vi "Scale.vi"(10 "Params":T1(array[cluster]), 11 "Frequences":dbl[](array[numeric])) -> (3 "ScaleFrequences":dbl[](array[numeric]))   [LabVIEW 2024]
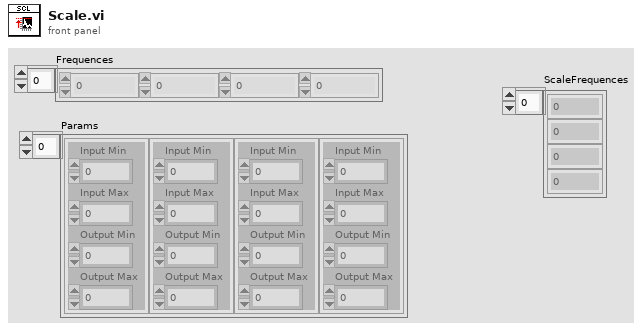
[diagram p1: front panel]
types:
  T1 = cluster{"Input Min":dbl, "Input Max":dbl, "Output Min":dbl, "Output Max":dbl}[]
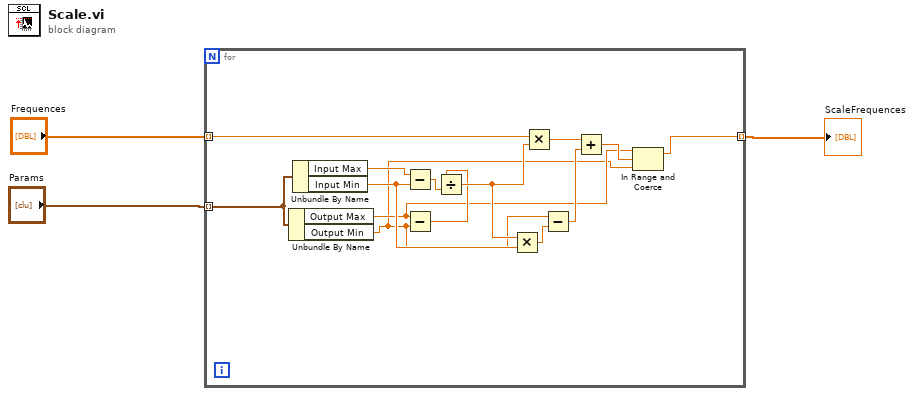
[diagram p0: block diagram]
diagram:
  n1 = for {
    tunnel: "Params" -> [w10] mode=indexing
    tunnel: "Frequences" -> [w11] mode=indexing
    tunnel: [w13] -> w1 mode=indexing
    n2 = Unbundle By Name(w10) -> ("Output Max"=w5:dbl, "Output Min"=w4:dbl)
    n3 = Unbundle By Name(w10) -> ("Input Max"=w12:dbl, "Input Min"=w6:dbl)
    n4 = Subtract(x=w12, y=w6) -> (x-y=w8:dbl)
    n5 = Subtract(x=w5, y=w4) -> (x-y=w7:dbl)
    n6 = Divide(x=w7, y=w8) -> (x/y=w9:dbl)
    n7 = Multiply(x=w9, y=w6) -> (x*y=w15:dbl)
    n8 = Multiply(x=w11, y=w9) -> (x*y=w17:dbl)
    n9 = Subtract(x=w4, y=w15) -> (x-y=w16:dbl)
    n10 = Add(x=w17, y=w16) -> (x+y=w14:dbl)
    n11 = In Range and Coerce(upper limit=w5, x=w14, lower limit=w4) -> (coerced(x)=w13:dbl)  [unwired: 1 out]
  }
  "ScaleFrequences" <- w1
